vi "GOMDBTS2048 get Handle.vi"(8 "error in (no error)":errorcluster, 11 "device":string) -> (0 "error out":errorcluster, 2 "function return":i32, 3 "handle":i32)   [LabVIEW 2015, in "GOMDBTS2048.lvlib"]
doc: "GOBTS2048DLL int __stdcall GOMDBTS2048_getHandle(char* device, int* handle);"
uses:
  GOMDBTS2048.lvlib
  runtime/GOMDBTS2048.dll
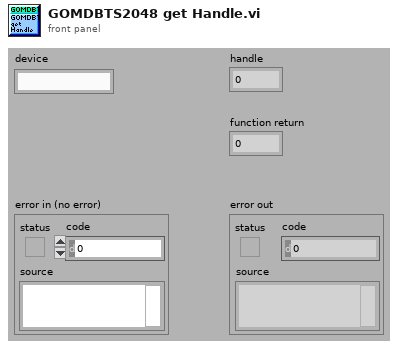
[diagram p1: front panel]
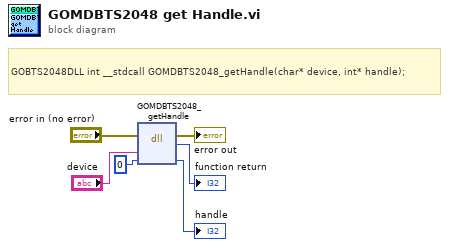
[diagram p0: block diagram]
diagram:
  # "GOBTS2048DLL int __stdcall GOMDBTS2048_getHandle(char* device, int* handle);"
  n1 = dll-call lib="C:/Users/rkoch/Documents/GO_Library/runtime/GOMDBTS2048.*" fn="GOMDBTS2048_getHandle"(error in="error in (no error)", "device"="device", "handle"=0) -> (error out=→"error out":errorcluster, →"function return":i32, "handle"=→"handle":i32)  [unwired: 3 in, 1 out]
